vi "Sim_Intake.vi"(11 "Motor Dmd":dbl) -> (3 "MotorRPM":dbl)   [LabVIEW 2023]
uses:
  <vilib>/Rock Robotics/WPI/ThirdParty/JAS_Junk/TrajLib/Enum/DCMOTOR_TYPES_ENUM.ctl
  <vilib>/Rock Robotics/WPI/ThirdParty/JAS_Junk/TrajLib/Trajectory_Library.lvlib
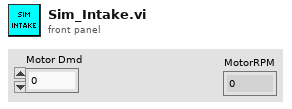
[diagram p1: front panel]
types:
  T1 = typedef "Trajectory_Library.lvlib/DCMOTOR_TYPES_ENUM.ctl" = enum16{"CIM", "AndyMark 9015", "Andy Mark RS 775 125", "Bag", "BaneBots RS 550", "BaneBots RS 775", "Falcon 500", "Mini CIM", "NEO", "NEO 550", "Romi BuiltIn", "Vex 775 Pro", "Snow Blower AM 2235A", "Bosch Seat AM 3493"}
  T2 = typedef "Trajectory_Library.lvlib/LINEAR_SYSTEM_ID_FLYWHEEL_MODEL.ctl" = cluster{"DCMOTOR_TYPES":T1, "Num Motors":i32, "Gearing":dbl, "MOI kgm2":dbl}
  T3 = typedef "Trajectory_Library.lvlib/FLYWHEEL_SIM_SIMULATION_PARAMS.ctl" = cluster{"Vel Meas Std Dev Rad/Sec":dbl}
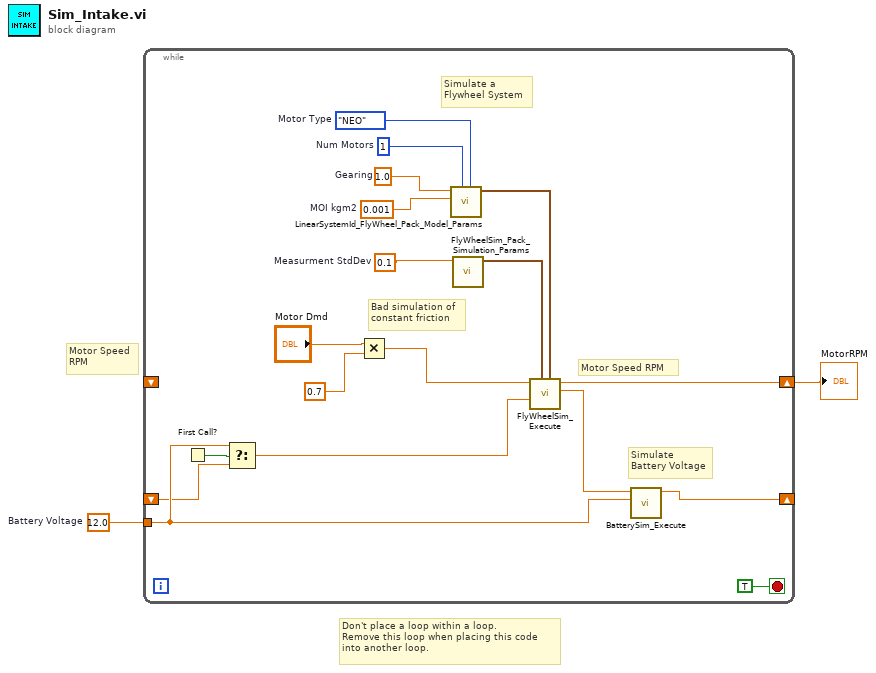
[diagram p0: block diagram]
diagram:
  w2 = 12.0  # Battery Voltage
  # "Don't place a loop within a loop. \nRemove this loop when placing this code\ninto another loop."
  # "Motor Speed\nRPM"
  n1 = while {
    shift-right: [w14] -> _
    shift-left: _ -> [w7]
    shift-right: [w13] -> w1
    shift-left: _ -> [_]
    tunnel: w2 -> [w8]
    stop <- TRUE stop-if-true
    w11 = 0.1  # Measurment StdDev
    w17 = 1.0  # Gearing
    w18 = 0.001  # MOI kgm2
    w19 = 1  # Num Motors
    w20 = DCMOTOR_TYPES_ENUM."NEO"  # Motor Type
    # "Bad simulation of\nconstant friction"
    # "Motor Speed RPM"
    # "Simulate\nBattery Voltage"
    # "Simulate a \nFlywheel System"
    n2 = First Call?() -> (First Call?: T/F=w9:bool)
    n3 = Select(t=w8, s=w9, f=w7) -> (s? t:f=w6:dbl)
    n4 = Multiply(x="Motor Dmd", y=0.7) -> (x*y=w4:dbl)
    n5 = call <vilib>:"LinearSystemId_FlyWheel_Pack_Model_Params.vi"("DCMOTOR_TYPES"=w20, "Num Motors"=w19, "MOI kgm2"=w18, "Gearing"=w17) -> ("LinearSystem_ID_FlyWheel_Model"=w12:T2)  [unwired: 7 in]
    n6 = call <vilib>:"FlyWheelSim_Pack_Simulation_Params.vi"("Vel Meas StdDev Rad/Sec"=w11) -> ("FlyWheelSim_Simulation_Params"=w10:T3)  [unwired: 10 in]
    n7 = call <vilib>:"FlyWheelSim_Execute.vi"("FlyWheelSim_Model _Params"=w12, "FlyWheelSim_Simulation_Params"=w10, "Battery Volts"=w6, "Motor Dmd"=w4) -> ("Motor Current"=w15:dbl, "Velocity_RPM"=w13:dbl)  [unwired: 4 in, 2 out]
    n8 = call <vilib>:"BatterySim_Execute.vi"("Nominal Battery Voltage"=w8, "Current"=w15) -> ("Voltage"=w14:dbl)  [unwired: 9 in]
  }
  "MotorRPM" <- w1
